vi "Example of SEQ.vi"() -> ()   [LabVIEW 2016]
uses:
  SEQ in variant.lvlib/SEQ.lvlib
panel:
  in  "stop":bool
  out "Data out":T1={"Refnum"=refnum, "Numeric"=4, "Array"=[]}
  in  "Data":T1={"Refnum"=refnum, "Numeric"=4, "Array"=[{"X"=1.0, "Y"=-1.0}]}
  out "error out":errorcluster
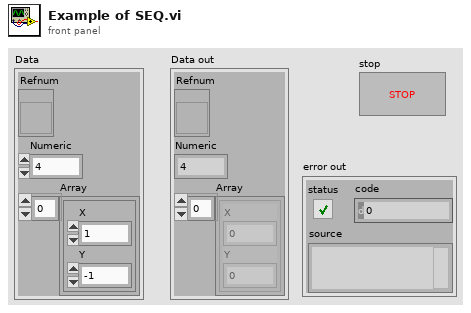
[diagram p1: front panel]
types:
  T1 = cluster{"Refnum":refnum<vi>, "Numeric":i32, "Array":cluster{"X":dbl, "Y":dbl}[]}
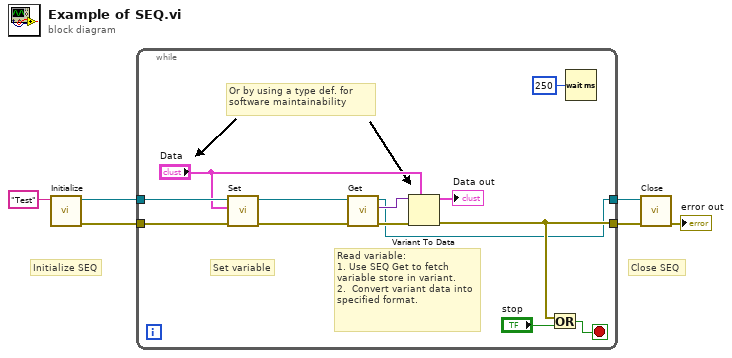
[diagram p0: block diagram]
diagram:
  # "Close SEQ"
  # "Initialize SEQ"
  n1 = call "Initialize.vi"("SEQ name"="Test") -> ("error out"=w3:errorcluster, "Ref out"=w5:refnum<queue>)  [unwired: 9 in]
  n2 = while {
    tunnel: w5 -> [w19]
    tunnel: [w7] -> w4
    tunnel: w3 -> [w17]
    tunnel: [w8] -> w2
    stop <- w14 stop-if-true
    # "Or by using a type def. for software maintainability"
    # "Read variable:\n1. Use SEQ Get to fetch variable store in variant.\n2.  Convert variant data into specified format."
    # "Set variable"
    n3 = call "Set.vi"("error in (no error)"=w17, "Variant"="Data", "Ref"=w19) -> ("error out"=w16:errorcluster, "Ref out"=w18:refnum<queue>)  [unwired: 7 in]
    n4 = call "Get.vi"("error in (no error)"=w16, "Ref"=w18) -> ("error out"=w9:errorcluster, "Variant"=w12:variant, "Ref out"=w7:refnum<queue>)  [unwired: 7 in]
    n5 = Variant To Data(error in=w9, type="Data", Variant=w12) -> (data=→"Data out":T1, error out=w8:errorcluster)
    n6 = Or(x=w8, y="stop") -> (x .or. y?=w14:bool)
    n7 = Wait (ms)(milliseconds to wait=u32 250) -> ()  [unwired: 1 out]
  }
  n8 = call "Close.vi"("error in (no error)"=w2, "Ref in"=w4) -> ("error out"=→"error out":errorcluster)  [unwired: 9 in]
